vi "RSMA Receiver - 3 SC 1 Channel.vi"() -> ()   [LabVIEW 2022 SP3]
panel:
  out "Iterations":dbl format="%#_4g"
  out "Number of bits":dbl[](array[numeric])
  out "Accuracy error":dbl[](array[numeric])
  out "Accumulated error":dbl[](array[numeric])
  in  "Decode M2?":bool
  out "Decoded Message - CH0":string
  out "Constellation Map":cdb[](graph)
  in  "Tab Control":enum32{"USRP Parameters", "Rx Info", "BER"}(tab)
  in  "USRP ControledParameters":T1={"Active Antenna"="RX2", "Gain (dB)"=0.0, "Carrier Frequency"=2400000000.0, "IQ Rate"=2000000.0, "Active channels"="0"} {"IQ Rate" format="%#_6p"; "Carrier Frequency" format="%#_6p"; "Gain (dB)" format="%#_6f"}
  in  "Device selection":refnum<k15>="RIO0"
  in  "Trigger level":dbl=0.01 format="%f"
  out "SIG valid?":bool
  out "Frequency offset":dbl
  out "Coerced Parameters":T2={"IQ Rate"=100000.0, "Carrier  Freq."=100000.0, "Gain"=0.0} {"Gain" format="%#_6f"; "Carrier  Freq." format="%#_6p"; "IQ Rate" format="%#_6p"}
  out "Error out":errorcluster
  in  "Expected message":string="Lorem ipsum dolor sit amet, consetetur sadipscing elitr, sed diam nonumy eirmod tempor invidunt ut labore et dolore magna aliquyam erat, sed diam volu"
  in  "Record BER":bool
  in  "Refresh Button":bool
  out "Inst. BER":dbl format="%#_4g"
  out "No. Bits":dbl format="%#_6f"
  out "Acum. Err":dbl
  out "Acc. BER":dbl format="%#_4g"
  in  "error in (no error)":errorcluster
  # "RSMA 3SC Receiver"
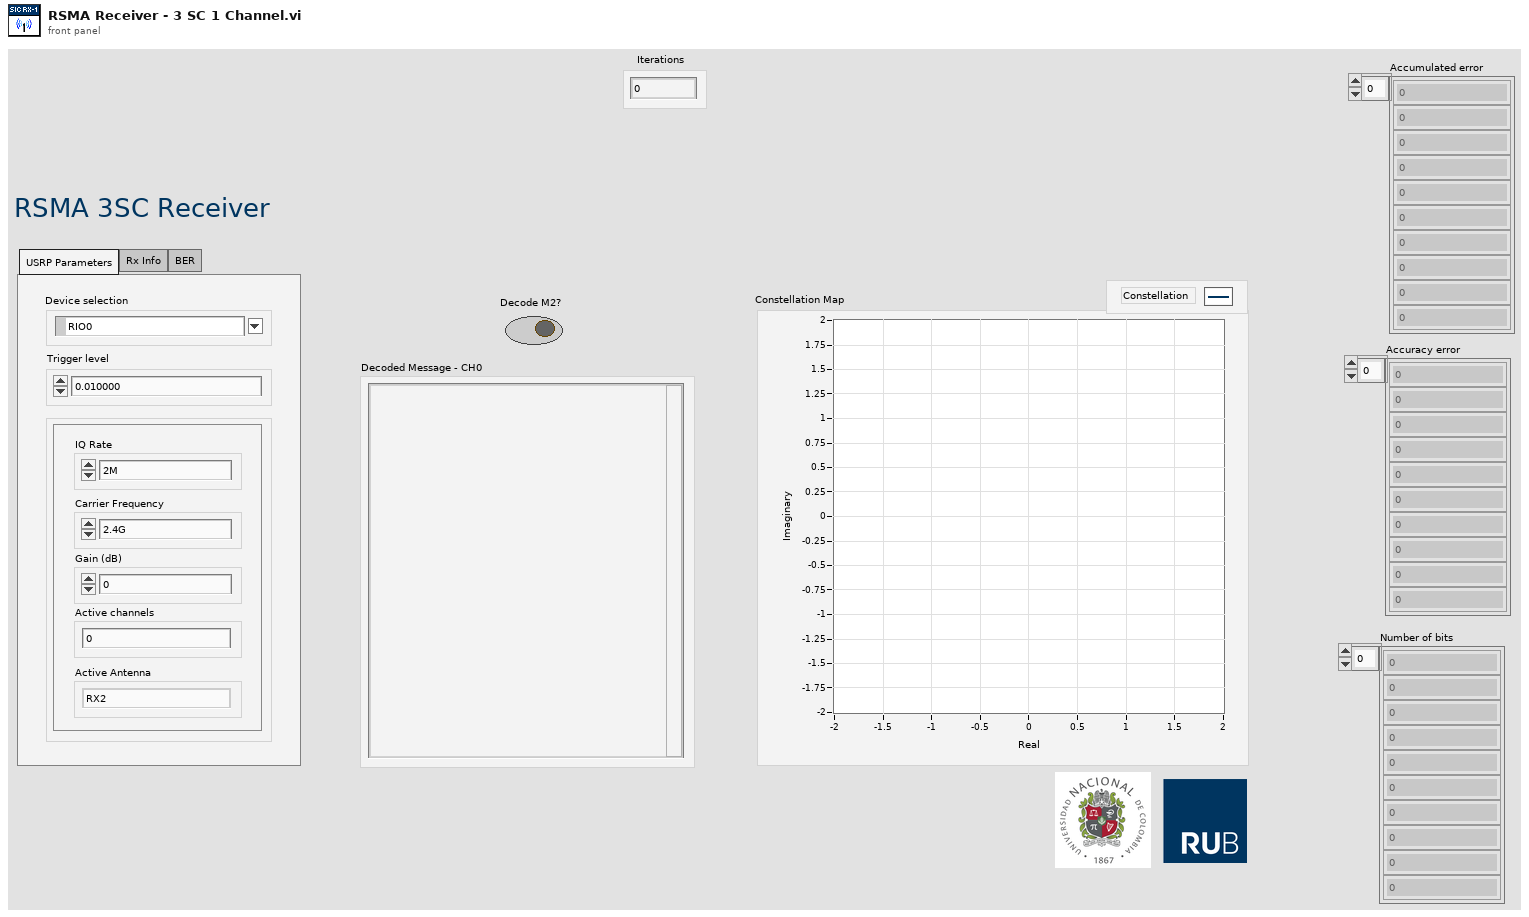
[diagram p1: front panel]
types:
  T1 = cluster{"Active Antenna":string, "Gain (dB)":dbl, "Carrier Frequency":dbl, "IQ Rate":dbl, "Active channels":string}
  T2 = cluster{"IQ Rate":dbl, "Carrier  Freq.":dbl, "Gain":dbl}
  T3 = cluster{"coerced IQ rate":dbl, "coerced carrier frequency":dbl, "coerced gain":dbl}
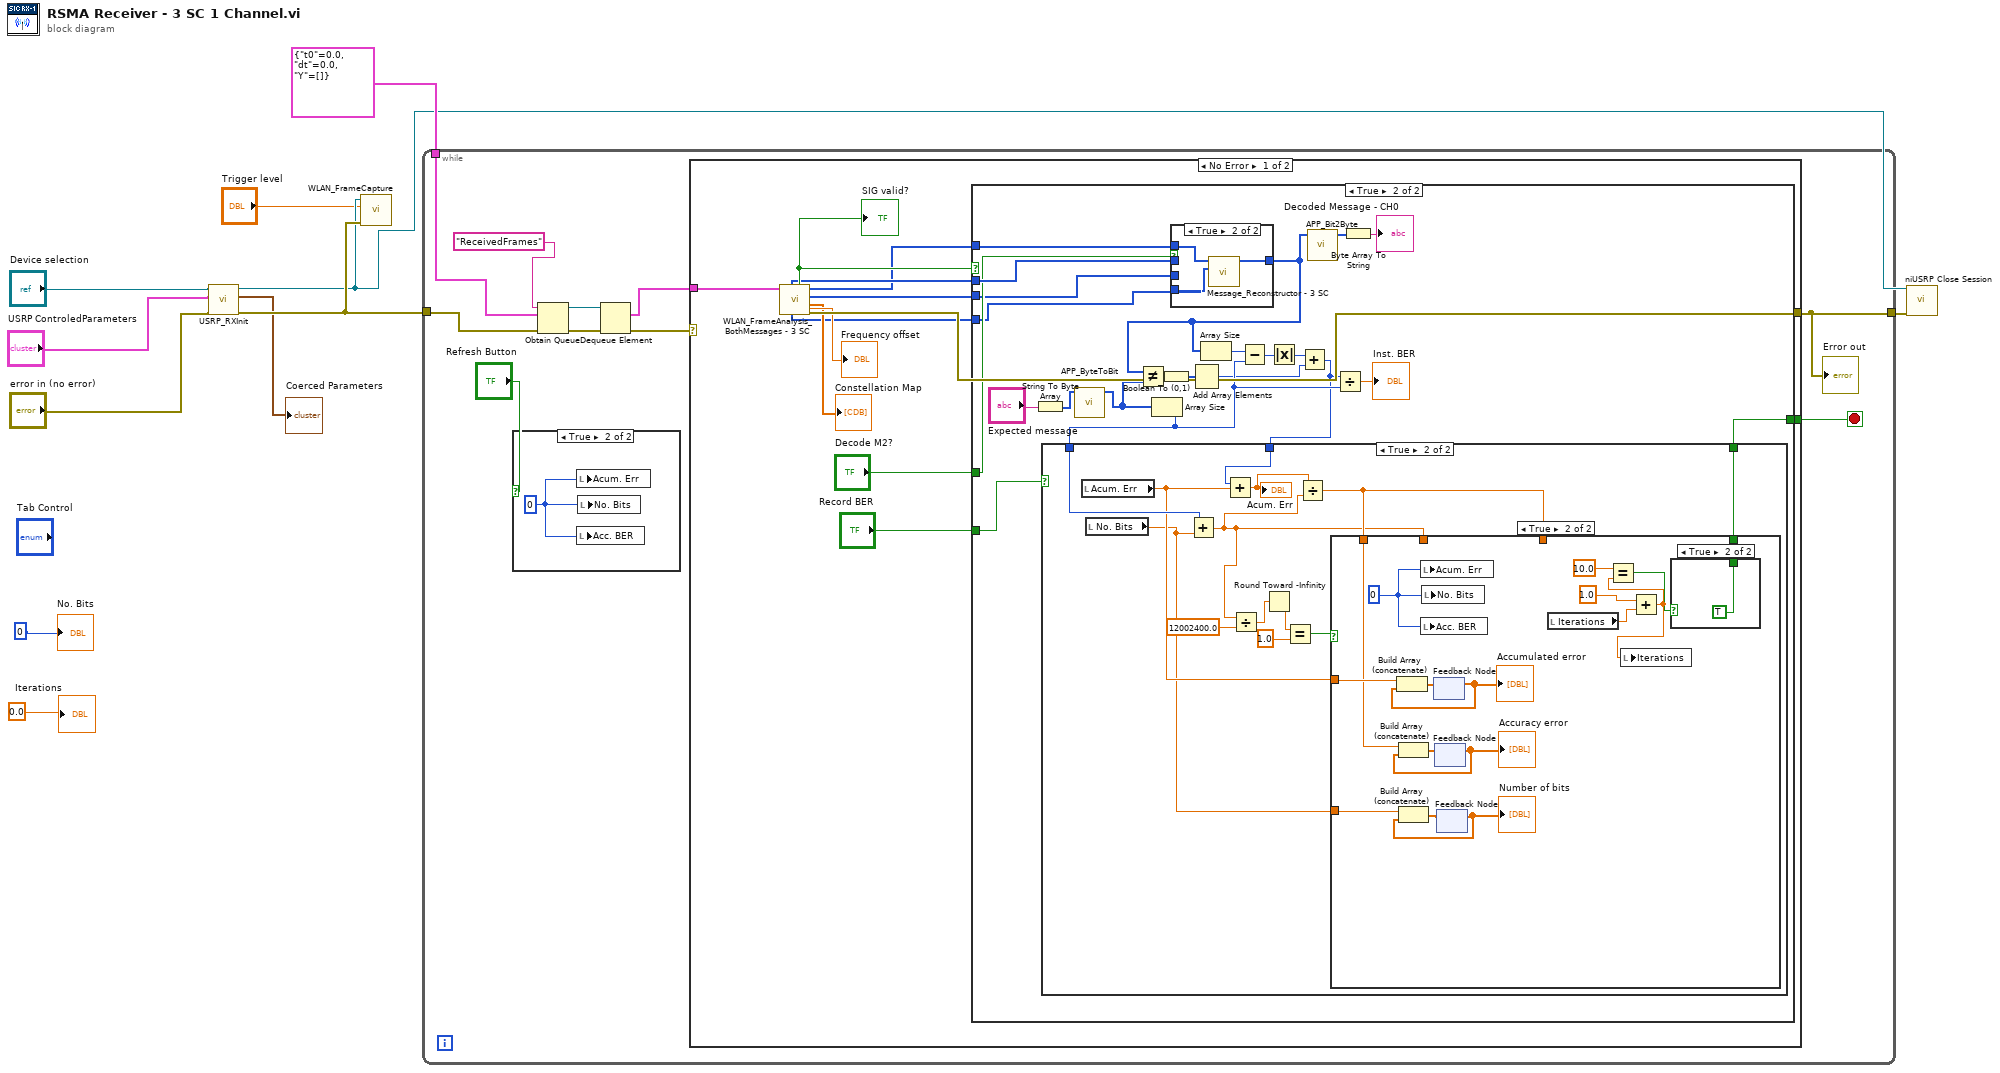
[diagram p0: block diagram]
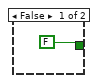
[diagram p3: hidden frame]
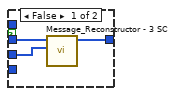
[diagram p4: hidden frame]
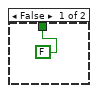
[diagram p5: hidden frame]
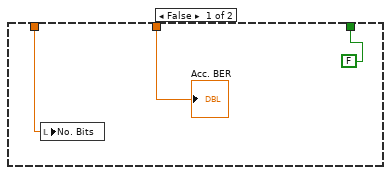
[diagram p6: hidden frame]
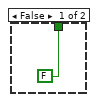
[diagram p7: hidden frame]
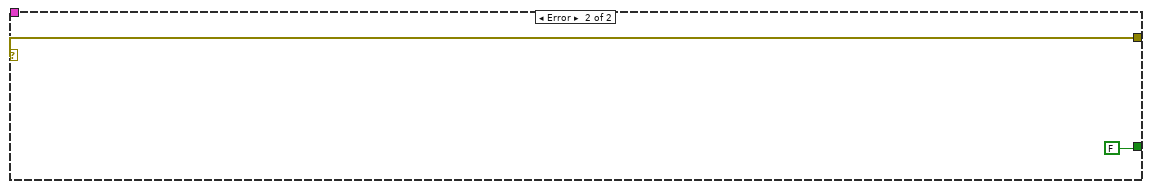
[diagram p8: hidden frame]
diagram:
  n1 = call "USRP_RXInit.vi"("device names"="Device selection", "USRP ControledParameters"="USRP ControledParameters", "error in (no error)"="error in (no error)") -> ("session handle out"=w7:refnum<k15>, "USRP CoercedParamters"=→"Coerced Parameters":T3, "error out"=w10:errorcluster)  [unwired: 5 in]
  n2 = call "WLAN_FrameCapture.vi"("error in (no error)"=w10, "Trigger level"="Trigger level", "session handle"=w7) -> ()  [unwired: 8 in]
  n3 = while {
    tunnel: w10 -> [w20]
    tunnel: cluster{"t0":dbl, "dt":dbl, "Y":cdb[]} {"t0"=0.0, "dt"=0.0, "Y"=[]} ("data") -> [w21]
    tunnel: [w14] -> w8
    stop <- w12 stop-if-true
    n4 = case shown="True" "Refresh Button" {
      frame False {
      }
      frame True {
        w22 = 0
        n5 = local write "Acum. Err"(w22) -> ()
        n6 = local write "Acc. BER"(w22) -> ()
        n7 = local write "No. Bits"(w22) -> ()
      }
    }
    n8 = Obtain Queue(name (unnamed)="ReceivedFrames", element data type=w21, error in (no error)=w20) -> (queue out=w19:refnum<queue>, error out=w16:errorcluster)  [unwired: 2 in, 1 out]
    n9 = Dequeue Element(queue=w19, error in (no error)=w16) -> (element=w17:cluster{"t0":dbl, "dt":dbl, "Y":cdb[]}, error out=w18:errorcluster)  [unwired: 1 in, 2 out]
    n10 = case shown="No Error" w18 {
      selector: w18 -> [_ w100]
      tunnel: w17 -> [w33 _]
      tunnel: [w34 w100] -> w14
      tunnel: [w23 FALSE] -> w12
      frame No Error {
        n11 = call "WLAN_FrameAnalysis_BothMessages - 3 SC.vi"("input cluster"=w33) -> ("error out"=w34:errorcluster, "Constellation"=→"Constellation Map":cdb[], "P1"=w25:i8[], "SC Bits"=w26:i8[], "Frequency offset"=→"Frequency offset":dbl, "SIG valid?"=w32:bool, "P2"=w24:i8[], "Base Bits"=w28:i8[])  [unwired: 3 in]
        "SIG valid?" <- w32
        n12 = case shown="True" w32 {
          tunnel: "Record BER" -> [_ w53]
          tunnel: w28 -> [_ w50]
          tunnel: "Decode M2?" -> [_ w40]
          tunnel: w26 -> [_ w39]
          tunnel: w25 -> [_ w38]
          tunnel: w24 -> [_ w37]
          tunnel: [FALSE w36] -> w23
          frame False {
          }
          frame True {
            n13 = String To Byte Array(string="Expected message") -> (unsigned byte array=w48:u8[])
            n14 = call "APP_ByteToBit.vi"("byte array"=w48) -> ("bit array"=w49:i8[])  [unwired: 9 in]
            n15 = Array Size(array=w49) -> (size(s)=w45:i32)
            n16 = case shown="True" w40 {
              tunnel: w38 -> [w58 _]
              tunnel: w50 -> [w59 _]
              tunnel: [w60 w63] -> w47
              tunnel: w37 -> [_ w61]
              tunnel: w39 -> [_ w62]
              frame False {
                n17 = call "Message_Reconstructor - 3 SC.vi"("Wp"=w58, "Wc"=w59) -> ("W1"=w60:u8[])  [unwired: 9 in]
              }
              frame True {
                n18 = call "Message_Reconstructor - 3 SC.vi"("Wp"=w61, "Wc"=w62) -> ("W1"=w63:u8[])  [unwired: 9 in]
              }
            }
            n19 = Not Equal?(x=w47, y=w49) -> (x != y?=w55:bool[])
            n20 = Boolean To (0,1)(Boolean=w55) -> (0, 1=w54:i16[])
            n21 = Add Array Elements(numeric array=w54) -> (sum=w42:i16)
            n22 = Array Size(array=w47) -> (size(s)=w46:i32)
            n23 = Subtract(x=w46, y=w45) -> (x-y=w44:i32)
            n24 = Absolute Value(x=w44) -> (abs(x)=w43:i32)
            n25 = Add(x=w43, y=w42) -> (x+y=w41:i32)
            n26 = case shown="True" w53 {
              tunnel: w45 -> [_ w77]
              tunnel: w41 -> [_ w76]
              tunnel: [FALSE w65] -> w36
              frame False {
              }
              frame True {
                n27 = local read "Acum. Err"() -> (w74:dbl)
                n28 = local read "No. Bits"() -> (w72:dbl)
                n29 = Add(x=w77, y=w72) -> (x+y=w71:dbl)
                n30 = Add(x=w76, y=w74) -> (x+y=w75:dbl)
                "Acum. Err" <- w75
                n31 = Divide(x=w71, y=12002400.0) -> (x/y=w69:dbl)
                n32 = Round Toward -Infinity(1:w69) -> (0:w67:dbl)
                n33 = Equal?(x=w67, y=1.0) -> (x = y?=w68:bool)
                n34 = Divide(x=w75, y=w71) -> (x/y=w73:dbl)
                n35 = case shown="True" w68 {
                  tunnel: w74 -> [_ w95]
                  tunnel: w71 -> [w80 _]
                  tunnel: w73 -> [w79 _]
                  tunnel: w73 -> [_ w92]
                  tunnel: w72 -> [_ w89]
                  tunnel: [FALSE w81] -> w65
                  frame False {
                    n36 = local write "No. Bits"(w80) -> ()
                    "Acc. BER" <- w79
                  }
                  frame True {
                    w96 = 0
                    n37 = local write "Acum. Err"(w96) -> ()
                    n38 = local write "Acc. BER"(w96) -> ()
                    n39 = local write "No. Bits"(w96) -> ()
                    n40 = feedback #1() -> (w93:dbl[])  [unwired: 1 in]
                    "Accumulated error" <- w93
                    n41 = Build Array (concatenate)(w95, w93) -> (w94:dbl[])
                    n42 = feedback-in #1(w94) -> ()
                    n43 = feedback #2() -> (w90:dbl[])  [unwired: 1 in]
                    "Accuracy error" <- w90
                    n44 = Build Array (concatenate)(w92, w90) -> (w91:dbl[])
                    n45 = feedback-in #2(w91) -> ()
                    n46 = feedback #3() -> (w87:dbl[])  [unwired: 1 in]
                    "Number of bits" <- w87
                    n47 = Build Array (concatenate)(w89, w87) -> (w88:dbl[])
                    n48 = feedback-in #3(w88) -> ()
                    n49 = local read "Iterations"() -> (w85:dbl)
                    n50 = Add(x=1.0, y=w85) -> (x+y=w82:dbl)
                    n51 = Equal?(x=10.0, y=w82) -> (x = y?=w83:bool)
                    n52 = local write "Iterations"(w82) -> ()
                    n53 = case shown="True" w83 {
                      tunnel: [FALSE TRUE] -> w81
                      frame False {
                      }
                      frame True {
                      }
                    }
                  }
                }
              }
            }
            n54 = call "APP_Bit2Byte.vi"("input bit stream"=w47) -> ("output byte stream"=w51:u8[])  [unwired: 10 in]
            n55 = Divide(x=w41, y=w45) -> (x/y=→"Inst. BER":dbl)
            n56 = Byte Array To String(unsigned byte array=w51) -> (string=→"Decoded Message - CH0":string)
          }
        }
      }
      frame Error {
      }
    }
    "Error out" <- w14
  }
  n57 = call <instrlib>:"niUSRP Close Session.vi"("session handle"=w7, "error in (no error)"=w8) -> ()  [unwired: 13 in, 1 out]
  "No. Bits" <- 0
  "Iterations" <- 0.0 ("Iterations")
